vi "Unsubscribe.vi"(7 "Time out (ms)":i32=1000, 8 "error in (no error)":errorcluster, 10 "Topic":string, 11 "WAMP Client in":refnum<class "WAMP Client.lvclass">) -> (0 "error out":errorcluster, 3 "WAMP Client out":refnum<class "WAMP Client.lvclass">)   [LabVIEW 2020, in "wamplv.lvlib" / "WAMP Client.lvclass"]
uses:
  WAMP Client.lvclass
  51763aff-f531-435e-9d49-62bb0d2b803c.vi
  TypeDefs/WAMP error.ctl
panel:
  out "WAMP Error":T1={"Details"="{}", "ArgumentKw Payload"="{}", "Error?"=FALSE, "Error URI"="", "Arguments Payload"=""}
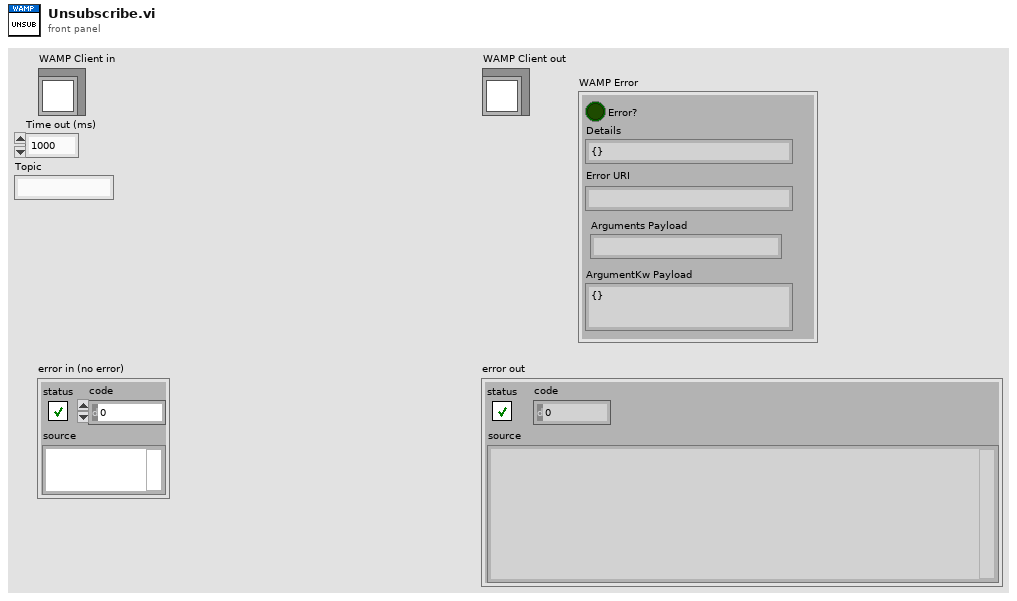
[diagram p1: front panel]
types:
  T1 = typedef "wamplv.lvlib/WAMP Client.lvclass/WAMP error.ctl" = cluster{"Details":string, "ArgumentKw Payload":string, "Error?":bool, "Error URI":string, "Arguments Payload":string}
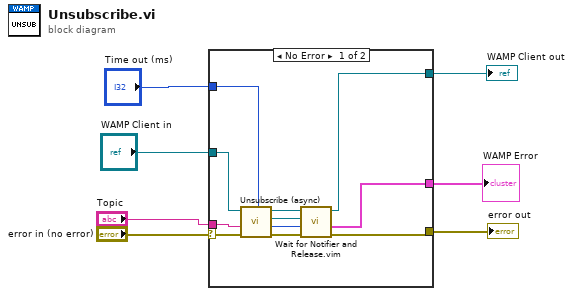
[diagram p0: block diagram]
diagram:
  n1 = case shown="No Error" "error in (no error)" {
    selector: "error in (no error)" -> [w16 w19]
    tunnel: [w13 w19] -> w7
    tunnel: [w9 w18] -> w5
    tunnel: "WAMP Client in" -> [w15 w18]
    tunnel: "Time out (ms)" -> [w8 _]
    tunnel: "Topic" -> [w17 _]
    tunnel: [w12 _] -> w1
    frame No Error {
      n2 = call-dynamic "Unsubscribe (async).vi"("error in (no error)"=w16, "Topic"=w17, "WAMP Client in"=w15) -> ("error out"=w14:errorcluster, "Result notifier"=w11:refnum<notifier>, "WAMP Client out"=w10:refnum<class "WAMP Client.lvclass">)  [unwired: 6 in]
      n3 = call "Wait for Notifier and Release.vim"("error in (no error)"=w14, "timeout in ms (-1)"=w8, "Notifier in"=w11, "WAMP Client in"=w10) -> ("error out"=w13:errorcluster, "WAMP Error"=w12:T1, "WAMP Client out"=w9:refnum<class "WAMP Client.lvclass">)  [unwired: 4 in, 1 out]
    }
    frame Error {
    }
  }
  "error out" <- w7
  "WAMP Client out" <- w5
  "WAMP Error" <- w1
